vi "hse-application_ApplicationInit.vi"(8 "error in":errorcluster, 10 "Project Folder":path, 11 "Project Name":string) -> (0 "error out":errorcluster)   [LabVIEW 2022 SP3, in "hse-application.lvclass"]
doc: "Initializes the HSE Application and its configuration variables with names, paths, version strings and other information.\n\n\n\n____\nHAMPEL SOFTWARE ENGINEERING v3.8.0 (2023-12-18 14:41)"
uses:
  hse-application.lvclass
  hse-misc/Controls/FGV_Actions.ctl
  hse-misc/hse-misc.lvlib
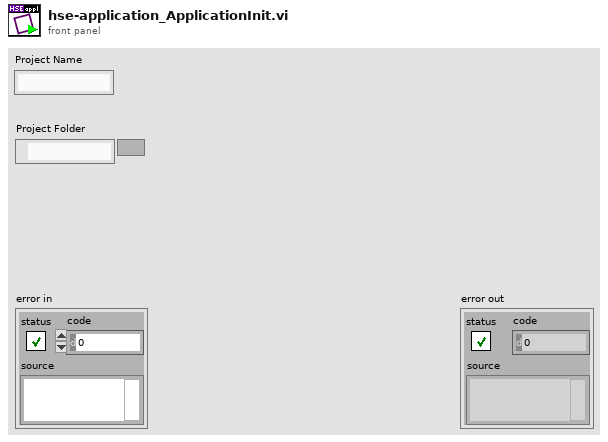
[diagram p1: front panel]
types:
  T1 = typedef "hse-misc.lvlib/FGV_Actions.ctl" = enum16{"Set", "Get"}
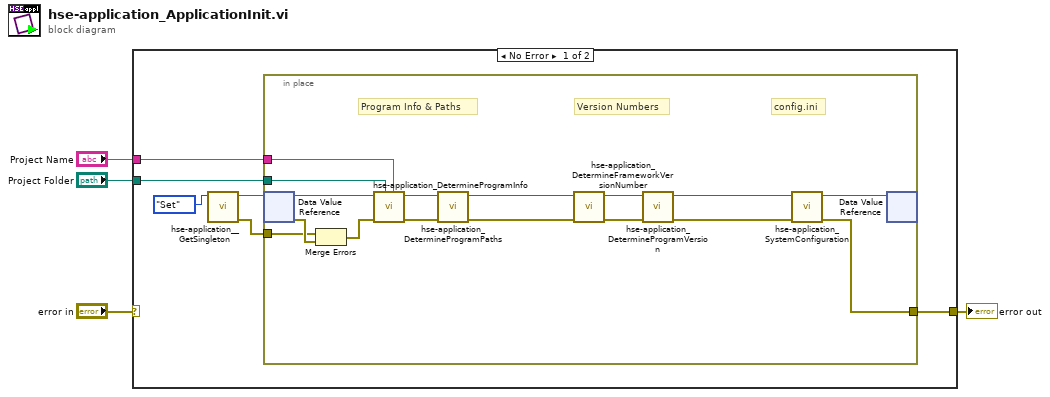
[diagram p0: block diagram]
diagram:
  n1 = case shown="No Error" "error in" {
    selector: "error in" -> [_ w27]
    tunnel: [w10 w27] -> w3
    tunnel: "Project Folder" -> [w8 _]
    tunnel: "Project Name" -> [w7 _]
    frame No Error {
      n2 = call "hse-application__GetSingleton.vi"("Action"=FGV_Actions."Set") -> ("Error Out"=w5:errorcluster, "ApplicationClass DVR"=w9:refnum<data-value>)  [unwired: 9 in]
      n3 = in-place "In Place Element Structure" {
        in-place-border: [w15] -> w10
        in-place-border: w8 -> [w14]
        in-place-border: w7 -> [w13]
        in-place-border: w5 -> [w11]
        # "config.ini"
        # "Version Numbers"
        # "Program Info & Paths"
        n4 = in-place-dvr #1(w9) -> (w24:refnum<class "hse-application.lvclass">, w23:errorcluster)
        n5 = Merge Errors(w11, w23) -> (w12:errorcluster)
        n6 = call "hse-application_DetermineProgramInfo.vi"("Project Name"=w13, "Project Folder"=w14, "error in"=w12, "Application in"=w24) -> ("error out"=w25:errorcluster, "Application out"=w26:refnum<class "hse-application.lvclass">)  [unwired: 6 in]
        n7 = call "hse-application_DetermineProgramPaths.vi"("error in"=w25, "Application in"=w26) -> ("error out"=w21:errorcluster, "Application out"=w22:refnum<class "hse-application.lvclass">)  [unwired: 8 in]
        n8 = call "hse-application_DetermineFrameworkVersionNumber.vi"("error in"=w21, "Application in"=w22) -> ("error out"=w19:errorcluster, "Application out"=w20:refnum<class "hse-application.lvclass">)  [unwired: 8 in]
        n9 = call "hse-application_DetermineProgramVersion.vi"("error in"=w19, "Application in"=w20) -> ("error out"=w18:errorcluster, "Application out"=w17:refnum<class "hse-application.lvclass">)  [unwired: 8 in]
        n10 = call "hse-application_SystemConfiguration.vi"("error in"=w18, "Application in"=w17) -> ("error out"=w15:errorcluster, "Application out"=w16:refnum<class "hse-application.lvclass">)  [unwired: 8 in]
        n11 = in-place-dvr #1(w16) -> ()  [unwired: 2 out]
      }
    }
    frame Error {
    }
  }
  "error out" <- w3
